vi "midiOutPlayer.msg.Stop.vi"(8 "error in (no error)":errorcluster, 11 "midiPlayer in":refnum<class "midiPlayer.lvclass">) -> (0 "error out":errorcluster, 3 "midiPlayer out":refnum<class "midiPlayer.lvclass">)   [LabVIEW 2020, in "midiPlayer.lvclass"]
uses:
  midiPlayer.lvclass
  midiPlayer.lvclass/midiPlayer.ctl
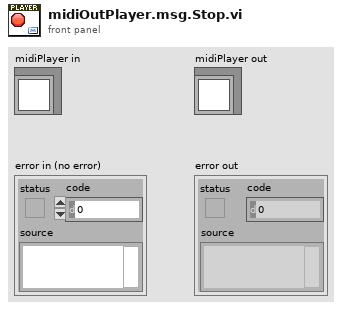
[diagram p1: front panel]
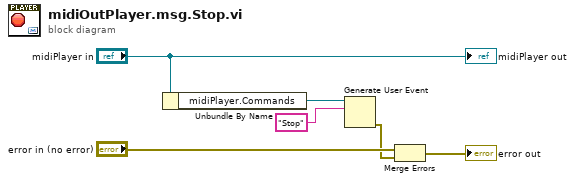
[diagram p0: block diagram]
diagram:
  n1 = Unbundle By Name("midiPlayer in") -> ("midiPlayer.Commands"=w6:refnum<user-event>)
  n2 = Generate User Event(user event=w6, event data cluster="Stop" ("event data")) -> (error out=w2:errorcluster)  [unwired: 2 in, 1 out]
  n3 = Merge Errors("error in (no error)", w2) -> (→"error out":errorcluster)
  "midiPlayer out" <- "midiPlayer in"
